vi "Write simulateSerialData.vi"(10 "simulateSerialData":refnum<class "SimulateSerialData.lvclass">, 11 "SerialSimulator in":refnum<class "SerialSimulator.lvclass">) -> (3 "SerialSimulator out":refnum<class "SerialSimulator.lvclass">)   [LabVIEW 2013, in "SerialProtocols.lvlib" / "SerialSimulator.lvclass"]
uses:
  <userlib>/Common/SerialProtocols/SerialProtocol/SerialSimulator/SerialSimulator.lvclass
  <userlib>/Common/Simulators/SimulateSerialData/SimulateSerialData.lvclass
  <userlib>/Common/SerialProtocols/SerialProtocol/SerialSimulator/SerialSimulator.lvclass/SerialSimulator.ctl
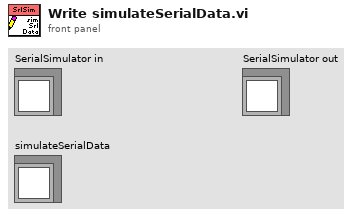
[diagram p1: front panel]
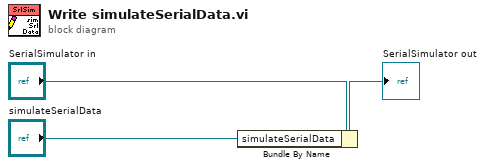
[diagram p0: block diagram]
diagram:
  n1 = Bundle By Name(cluster="SerialSimulator in", "simulateSerialData"="simulateSerialData") -> (→"SerialSimulator out":refnum<class "SerialSimulator.lvclass">)
